vi "program_supply2.vi"() -> ()   [LabVIEW 2018]
uses:
  <vilib>/MakerHub/LINX/Public/Peripherals/PWM/PWM Set Duty Cycle 1 Chan.vi
  <vilib>/MakerHub/LINX/Public/Utilities/Open Serial.vi
  <vilib>/MakerHub/LINX/Public/Peripherals/PWM/PWM Set Duty Cycle N Chans.vi
  <vilib>/MakerHub/LINX/LMH-LINX.lvlib
panel:
  in  "Serial Port":refnum<visa-resource-name>="N/A"
  in  "File Name":string
  in  "停止":bool
  in  "File Path":path
  in  "通道六（V）":dbl
  in  "通道五（V）":dbl
  in  "通道四（V）":dbl
  in  "通道三（V）":dbl
  in  "通道二（V）":dbl
  in  "通道一（V）":dbl
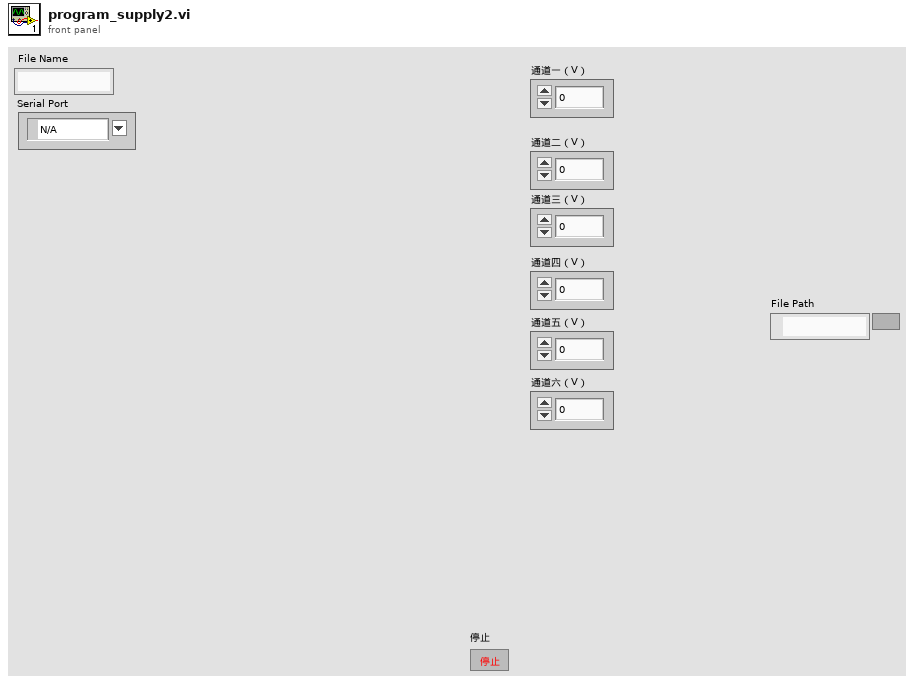
[diagram p1: front panel]
types:
  T1 = enum16{"open", "replace", "create", "open or create", "replace or create", "replace or create with confirmation"}
  T2 = typedef "LMH-LINX.lvlib/LINX Ref.ctl" = cluster{"IO":T3, "Interface":T4, "LINX Device Config":T5}
  T3 = typedef "LMH-LINX.lvlib/Platform.ctl" = enum16{"Remote", "Local"}
  T4 = typedef "LMH-LINX.lvlib/Interface.ctl" = enum16{"Serial", "TCP"}
  T5 = typedef "LMH-LINX.lvlib/Device.lvlib/LINX Device Config.ctl" = cluster{"Interface":T4, "COM Port":refnum<visa-resource-name>, "TCP Configuration":T6, "Device Family":u8, "Device ID":u8, "Device Name":string, "TCP Ref":refnum<k5>, "Channels":T7}
  T6 = typedef "LMH-LINX.lvlib/Device.lvlib/TCP Config.ctl" = cluster{"IP Address":string, "Port":u16}
  T7 = typedef "LMH-LINX.lvlib/Channels.ctl" = cluster{"DI":u8[], "DO":u8[], "AI":u8[], "AO":u8[], "PWM":u8[], "QE":u8[], "UART":u8[], "I2C 2":u8[], "SPI":u8[], "CAN":u8[], "Servo":u8[], "AI Ref (V)":dbl, "AI Resolution (Bits)":u8, "AO Ref (V)":dbl, "AO Resolution (Bits)":u8}
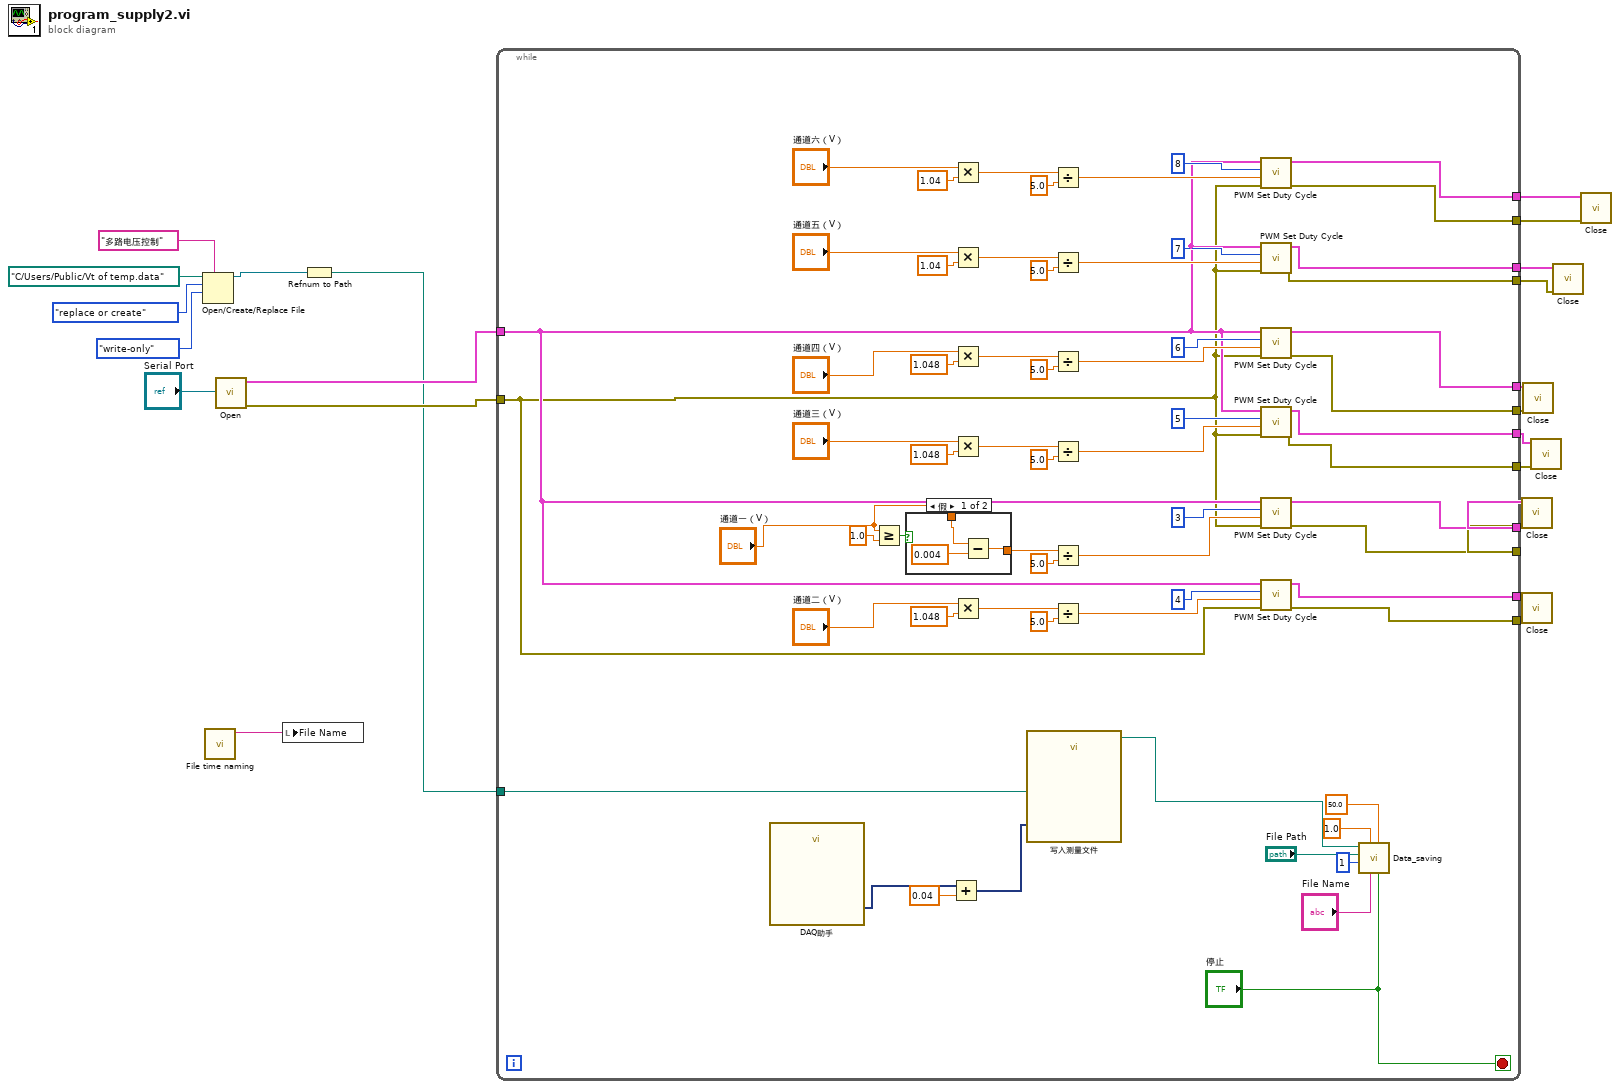
[diagram p0: block diagram]
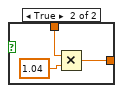
[diagram p2: hidden frame]
diagram:
  n1 = Open/Create/Replace File(file path (use dialog)=path "C:/Users/Public/Vt of temp.data" ("文件路径（使用对话框）"), prompt="多路电压控制" ("提示"), operation (0:open)=T1."replace or create" ("操作(0:open)"), access (0:read/write)=enum16{"read/write", "read-only", "write-only"}."write-only" ("权限(0:read/write)")) -> (refnum out=w4:refnum<file>)  [unwired: 2 in, 2 out]
  n2 = call "File time naming.vi"() -> ("result string"=w3:string)  [unwired: 11 in]
  n3 = call-poly <vilib>:"Open.vi"("Serial Port"="Serial Port") -> ("Error Out"=w17:errorcluster, "LINX Resource"=w18:T2)  [unwired: 8 in, 1 out]
  n4 = local write "File Name"(w3) -> ()
  n5 = Refnum to Path(1:w4) -> (0:w2:path)
  n6 = while {
    tunnel: w18 -> [w50]
    tunnel: w17 -> [w49]
    tunnel: [w48] -> w16
    tunnel: [w47] -> w15
    tunnel: [w46] -> w14
    tunnel: [w45] -> w13
    tunnel: [w44] -> w12
    tunnel: [w43] -> w11
    tunnel: [w42] -> w10
    tunnel: [w41] -> w9
    tunnel: [w40] -> w8
    tunnel: [w39] -> w7
    tunnel: [w38] -> w6
    tunnel: [w37] -> w5
    tunnel: w2 -> [w29]
    stop <- "停止" stop-if-true
    n7 = call "DAQ助手"() -> ("data"=w28:dynamicdata)  [unwired: 16 in, 3 out]
    n8 = Greater Or Equal?(x="通道一（V）", y=1.0) -> (x >= y?=w23:bool)
    n9 = case shown="假" w23 {
      tunnel: [w87 w89] -> w83
      tunnel: "通道一（V）" -> [w86 w88]
      frame False {
        n10 = Subtract(x=w86, y=0.004) -> (x-y=w87:dbl)
      }
      frame True {
        n11 = Multiply(x=w88, y=1.04) -> (x*y=w89:dbl)
      }
    }
    n12 = Add(x=w28, y=0.04) -> (x+y=w26:dynamicdata)
    n13 = Multiply(x="通道六（V）", y=1.04) -> (x*y=w59:dbl)
    n14 = Multiply(x="通道五（V）", y=1.04) -> (x*y=w63:dbl)
    n15 = Multiply(x="通道四（V）", y=1.048) -> (x*y=w67:dbl)
    n16 = Multiply(x="通道三（V）", y=1.048) -> (x*y=w71:dbl)
    n17 = Multiply(x="通道二（V）", y=1.048) -> (x*y=w76:dbl)
    n18 = call "写入测量文件"("Signals"=w26, "Filename"=w29) -> ("Filename Out"=w32:path)  [unwired: 15 in, 2 out]
    n19 = Divide(x=w59, y=5.0) -> (x/y=w55:dbl)
    n20 = Divide(x=w63, y=5.0) -> (x/y=w56:dbl)
    n21 = Divide(x=w67, y=5.0) -> (x/y=w57:dbl)
    n22 = Divide(x=w71, y=5.0) -> (x/y=w58:dbl)
    n23 = Divide(x=w83, y=5.0) -> (x/y=w82:dbl)
    n24 = Divide(x=w76, y=5.0) -> (x/y=w75:dbl)
    n25 = call-poly <vilib>:"PWM Set Duty Cycle.vi"("Error In"=w49, "Duty Cycle (0-1)"=w55, "PWM Channel"=u8 8, "LINX Resource"=w50) -> ("Error Out"=w47:errorcluster, "LINX Resource"=w48:T2)  [unwired: 6 in]
    n26 = call-poly <vilib>:"PWM Set Duty Cycle.vi"("Error In"=w49, "Duty Cycle (0-1)"=w56, "PWM Channel"=u8 7, "LINX Resource"=w50) -> ("Error Out"=w45:errorcluster, "LINX Resource"=w46:T2)  [unwired: 6 in]
    n27 = call-poly <vilib>:"PWM Set Duty Cycle.vi"("Error In"=w49, "Duty Cycle (0-1)"=w57, "PWM Channel"=u8 6, "LINX Resource"=w50) -> ("Error Out"=w43:errorcluster, "LINX Resource"=w44:T2)  [unwired: 6 in]
    n28 = call-poly <vilib>:"PWM Set Duty Cycle.vi"("Error In"=w49, "Duty Cycle (0-1)"=w58, "PWM Channel"=u8 5, "LINX Resource"=w50) -> ("Error Out"=w41:errorcluster, "LINX Resource"=w42:T2)  [unwired: 6 in]
    n29 = call-poly <vilib>:"PWM Set Duty Cycle.vi"("Error In"=w49, "Duty Cycle (0-1)"=w82, "PWM Channel"=u8 3, "LINX Resource"=w50) -> ("Error Out"=w39:errorcluster, "LINX Resource"=w40:T2)  [unwired: 6 in]
    n30 = call-poly <vilib>:"PWM Set Duty Cycle.vi"("Error In"=w49, "Duty Cycle (0-1)"=w75, "PWM Channel"=u8 4, "LINX Resource"=w50) -> ("Error Out"=w37:errorcluster, "LINX Resource"=w38:T2)  [unwired: 6 in]
    n31 = call "Data_saving.vi"("Boolean"="停止", "Sampling Rate"=50.0, "File Name"="File Name", "Voltage Sensitivity\n1000 will be 1000"=1.0 ("Voltage Sensitivity\n1000 will be 1000"), "Number of Samples Per Channel"=1, "File Path"="File Path", "File name source"=w32) -> ()  [unwired: 5 in]
  }
  n32 = call <vilib>:"Close.vi"("Error In"=w7, "LINX Resource"=w8) -> ()  [unwired: 9 in, 1 out]
  n33 = call <vilib>:"Close.vi"("Error In"=w5, "LINX Resource"=w6) -> ()  [unwired: 9 in, 1 out]
  n34 = call <vilib>:"Close.vi"("Error In"=w11, "LINX Resource"=w12) -> ()  [unwired: 9 in, 1 out]
  n35 = call <vilib>:"Close.vi"("Error In"=w9, "LINX Resource"=w10) -> ()  [unwired: 9 in, 1 out]
  n36 = call <vilib>:"Close.vi"("Error In"=w13, "LINX Resource"=w14) -> ()  [unwired: 9 in, 1 out]
  n37 = call <vilib>:"Close.vi"("Error In"=w15, "LINX Resource"=w16) -> ()  [unwired: 9 in, 1 out]
